vi "看板状态.vi"(8 "错误输入（无错误）":errorcluster, 10 "附加信息":string, 11 "设备状态":enum16{"设备离线", "设备正常", "设备缺料", "设备故障", "质量报警"}(ring)=enum."设备正常") -> (0 "错误输出":errorcluster)   [LabVIEW 2020]
uses:
  Global1.vi
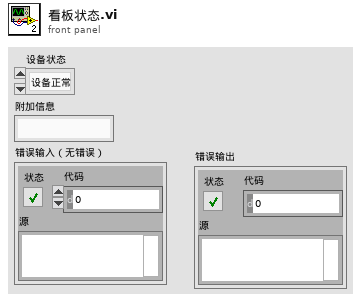
[diagram p1: front panel]
types:
  T1 = cluster{"设备名称":string, "操作人员":string, "设备状态":enum16{"设备离线", "设备正常", "设备缺料", "设备故障", "质量报警"}, "附加信息":string}
  T2 = cluster{"用户编号":string, "用户名":string, "用户密码(密文)":string, "用户权限":string}
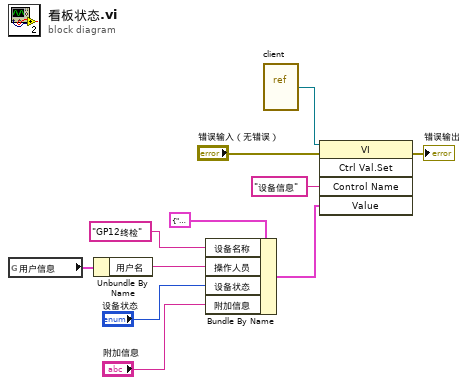
[diagram p0: block diagram]
diagram:
  n1 = global read "Global1.vi" "用户信息"() -> (w9:T2)
  n2 = Unbundle By Name(w9) -> ("用户名"=w6:string)
  n3 = Bundle By Name(cluster=T1 {"设备名称"="", "操作人员"="", "设备状态"=enum."设备正常", "附加信息"=""} ("设备信息"), "设备名称"="GP12终检", "操作人员"=w6, "设备状态"="设备状态", "附加信息"="附加信息") -> (w3:T1)
  n4 = vi-ref "client.vi"() -> (w11:refnum<vi>)
  n5 = invoke class="VI" method="Ctrl Val.Set"(reference=w11, error in="错误输入（无错误）", "Control Name"="设备信息" ("控件名"), "Value"=w3) -> (error out=→"错误输出":errorcluster)  [unwired: 1 in, 4 out]
